vi "Get Ac Dc.vi"(11 "channel":u32) -> (3 "function return":i32)   [LabVIEW 2021, in "vmmso.lvlib"]
doc: "DLL_API int WINAPI GetAcDc(unsigned int channel);"
uses:
  vmmso.lvlib
  vmmso.dll
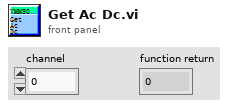
[diagram p1: front panel]
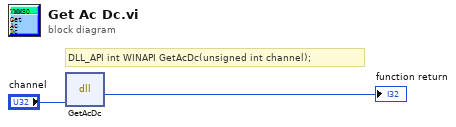
[diagram p0: block diagram]
diagram:
  # "DLL_API int WINAPI GetAcDc(unsigned int channel);"
  n1 = dll-call lib="D:/labviewdemo/LabviewDemo 21/vmmso/vmmso.*" fn="GetAcDc"("channel"="channel") -> (→"function return":i32)  [unwired: 4 in, 2 out]
